vi "FlashModel.vi"() -> ()   [LabVIEW 2013]
uses:
  GlobalV.vi
panel:
  in  "取消":bool
  in  "确定":bool
  in  "型号":u16(ring) caption="产品原始型号" items=["90-18", "90-68"]
  out "Result":bool
  in  "新的型号值":string
  out "ArrayOut":string[](array[string])
  in  "条码内容":string
  # "注意刷新部分产品型号之后，请在配置文件BSJ.ini\n中添加新型号的配置参数，刷新前请先选中产品的\n原始型号"
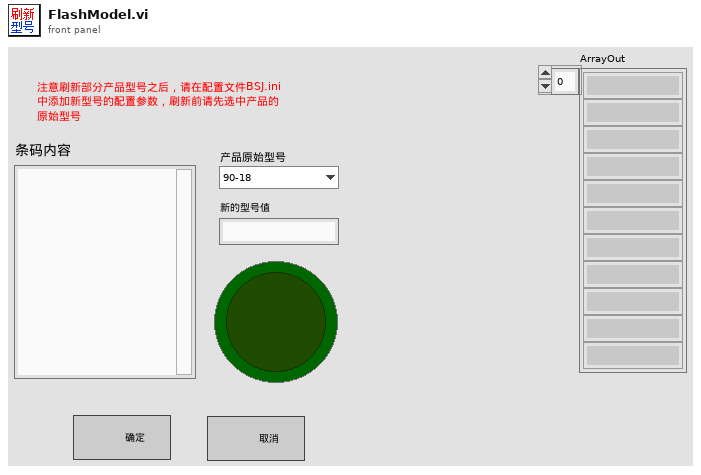
[diagram p1: front panel]
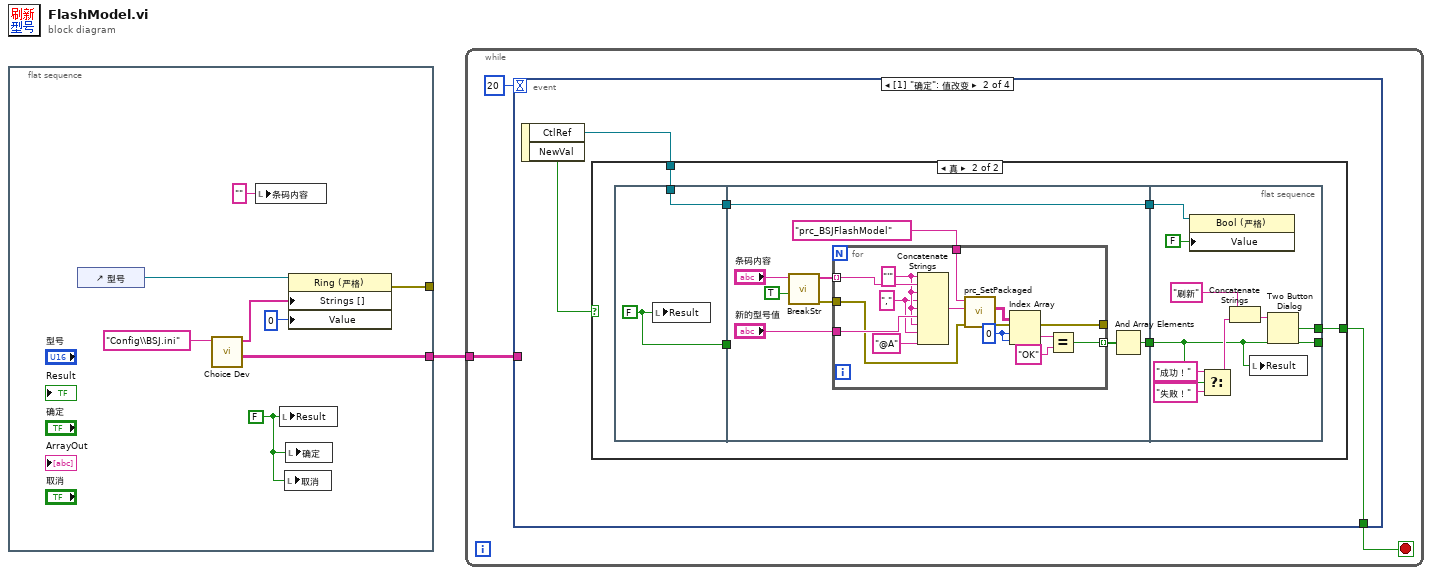
[diagram p0: block diagram]
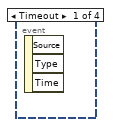
[diagram p2: hidden frame]
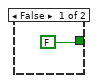
[diagram p3: hidden frame]
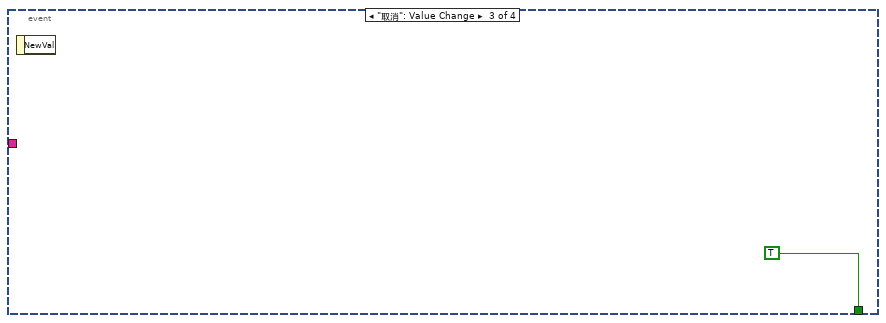
[diagram p4: hidden frame]
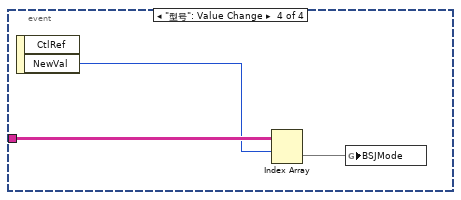
[diagram p5: hidden frame]
diagram:
  n1 = flat-sequence {
    tunnel: [w8] -> w1
    tunnel: [w4] -> _
    frame #0 {
      w3 = FALSE
      n2 = control-ref of="型号"() -> (w7:refnum<vi>)
      n3 = call "Choice Dev.vi"("Path"="Config\\BSJ.ini") -> ("data"=w8:string[][], "model"=w6:string[])  [unwired: 7 in, 1 out]
      n4 = local write "条码内容"("" ("条码内容")) -> ()
      n5 = local write "Result"(w3) -> ()
      n6 = local write "取消"(w3) -> ()
      n7 = local write "确定"(w3) -> ()
      n8 = property class="Ring (严格)"(reference=w7, "Strings []"=w6, "Value"=0) -> (error out=w4:errorcluster)  [unwired: 1 in, 1 out]
    }
  }
  n9 = while {
    tunnel: w1 -> [w11]
    stop <- w10 stop-if-true
    n10 = event shown="[1] \"确定\": 值改变" {
      selector: _ -> [_ _ _ _]
      dyn-events: _ -> [_ _ _ _]
      timeout: 20 -> [_ _ _ _]
      tunnel: w11 -> [_ _ _ w60]
      tunnel: [_ w15 TRUE _] -> w10
      event Timeout {
        n11 = event-data() -> ()  [unwired: 1 in, 3 out]
      }
      event "确定": Value Change {
        n12 = event-data() -> ("CtlRef"=w14:refnum<vi>, "NewVal"=w13:bool)  [unwired: 1 in]
        n13 = case shown="真" w13 {
          tunnel: [FALSE w18] -> w15
          tunnel: w14 -> [_ w17]
          frame False {
          }
          frame True {
            n14 = flat-sequence {
              tunnel: [w24] -> w22
              tunnel: [w23] -> w21
              tunnel: w17 -> [w23]
              tunnel: w22 -> [_]
              tunnel: [w26] -> w20
              tunnel: [w25] -> w19
              tunnel: w21 -> [w25]
              tunnel: [w51] -> _
              tunnel: w20 -> [w51]
              tunnel: [w55] -> w18
              tunnel: w19 -> [w49]
              frame #0 {
                w24 = FALSE
                n15 = local write "Result"(w24) -> ()
              }
              frame #1 {
                n16 = call "BreakStr.vi"("外购？"=TRUE, "StrIn"="条码内容") -> ("error out"=w28:errorcluster, "ArrayOut"=w30:string[])  [unwired: 8 in]
                n17 = for {
                  tunnel: "prc_BSJFlashModel" ("SQL query") -> [w47]
                  tunnel: w30 -> [w45] mode=indexing
                  tunnel: "新的型号值" -> [w44]
                  tunnel: w28 -> [w40]
                  tunnel: [w39] -> _
                  tunnel: [w34] -> w27 mode=indexing
                  w37 = 0
                  w42 = ","
                  w43 = "'"
                  n18 = Concatenate Strings(w43, w45, w43, w42, w43, w44, w43, w42, "@A") -> (w46:string)
                  n19 = call "prc_SetPackaged.vi"("error in"=w40, "string"=w46, "SQL query"=w47) -> ("error out"=w39:errorcluster, "Array"=w38:string[][])  [unwired: 7 in]
                  n20 = Index Array(array=w38, index (row)=w37, index (col)=w37) -> (element=w36:string)
                  n21 = Equal?(x=w36, y="OK") -> (x = y?=w34:bool)
                }
                n22 = And Array Elements(Boolean array=w27) -> (logical AND=w26:bool)
              }
              frame #2 {
                n23 = property class="Bool (严格)"(reference=w49, "Value"=FALSE) -> ()  [unwired: 1 in, 2 out]
                n24 = Select(t="成功！" ("消息"), s=w51, f="失败！" ("消息")) -> (s? t:f=w52:string)
                n25 = Concatenate Strings("刷新" ("消息"), w52) -> (w54:string)
                n26 = local write "Result"(w51) -> ()
                n27 = Two Button Dialog(message=w54) -> (T button?=w55:bool)  [unwired: 2 in]
              }
            }
          }
        }
      }
      event "取消": Value Change {
        n28 = event-data() -> ()  [unwired: 1 in, 1 out]
      }
      event "型号": Value Change {
        n29 = event-data() -> ("NewVal"=w59:u16)  [unwired: 1 in, 1 out]
        n30 = Index Array(array=w60, index (row)=w59) -> (element=w58:string[])  [unwired: 1 in]
        n31 = global write "GlobalV.vi" "BSJMode"(w58) -> ()
      }
    }
  }
